vi "BRAM.vi"() -> ()   [LabVIEW 2011]
uses:
  <vilib>/rvi/IPIntegrationNode/IPINode_Utilities/niFpgaIPINodeSimCore.vi
  <vilib>/rvi/XilinxIP/XIPIN_XNode/niFpgaXIPIN.xnode
  <userlib>/FPGA Library/Code Development/Signal Processing/FFT/Real Sequence from Complex FFT/BRAMCore/Block_Memory_Generator_968CC79E400EC6543E31E683AFFB55E2.dll
  <vilib>/rvi/IPIntegrationNode/IPINode_Xnode/niFpgaIPINode.xnode
panel:
  out "doutb":fxp<+,16,16>
  out "douta":fxp<+,16,16>
  in  "dinb":fxp<+,16,16>
  in  "addrb":fxp<+,4,4>
  in  "dina":fxp<+,16,16>
  in  "addra":fxp<+,4,4>
  in  "wea":bool
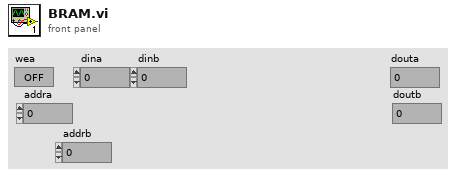
[diagram p1: front panel]
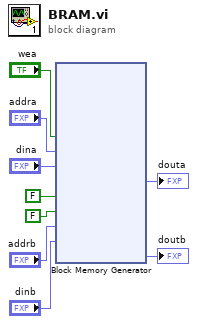
[diagram p0: block diagram]
diagram:
  n1 = xnode ("Block Memory Generator")("wea"="wea", "addra"="addra", "dina"="dina", "clkb"=FALSE, "web"=FALSE, "addrb"="addrb", "dinb"="dinb") -> ("douta"=→"douta":fxp<+,16,16>, "doutb"=→"doutb":fxp<+,16,16>)
